vi "Read Core OOB TX.vi"(8 "error in (no error)":errorcluster, 11 "CIFCorePlugin in":refnum<class "CIFCorePlugin.lvclass">) -> (0 "error out":errorcluster, 3 "CIFCorePlugin out":refnum<class "CIFCorePlugin.lvclass">)   [LabVIEW 2021, in "CIFCorePlugin.lvclass"]
uses:
  CIFCorePlugin.lvclass
  CIFCorePlugin.lvclass/CIFCorePlugin.ctl
  Channels/CIFChannelMng/CIFChannelMng.lvclass/CIFChannelMng.ctl
  e064c0da-9abb-41e4-9ae5-21a8637ddf9c.vi
  Channels/CIFChannelMng/SubVIs/Read Channel List.vi
  Channels/CIFChannelMng/Core/Refresh Channel Data.vi/8bba354e-317d-4116-a685-ab5cd7060b87.vi
  <vilib>/CIF Foundation/CIF CIPC/SubVIs/Wait For N Elements Available.vi
  <vilib>/CIF Foundation/CIF CIPC/SubVIs/Check Error.vi
  <vilib>/CIF Foundation/CIF CIPC/SubVIs/Get dll Path.vi
  <vilib>/CIF Foundation/CIF CIPC/SubVIs/Get Element Read Position.vi
  <vilib>/CIF Foundation/CIF CIPC/SubVIs/Set Element Read Position.vi
  Utilities/Clocks/Update Clock.vi
  <vilib>/CIF Foundation/CIF CIPC/SubVIs/Get Element Info Variant.vi
  <vilib>/Utility/error.llb/Trim Whitespace.vi
  <vilib>/Utility/error.llb/Error Cluster From Error Code.vi
  CIFPluginManager/gRPC/CIF_Manager_Client_Wrapper/Internal/Update Clock.vi
  Channels/CIFChannelMng/CIFChannelMng.lvclass
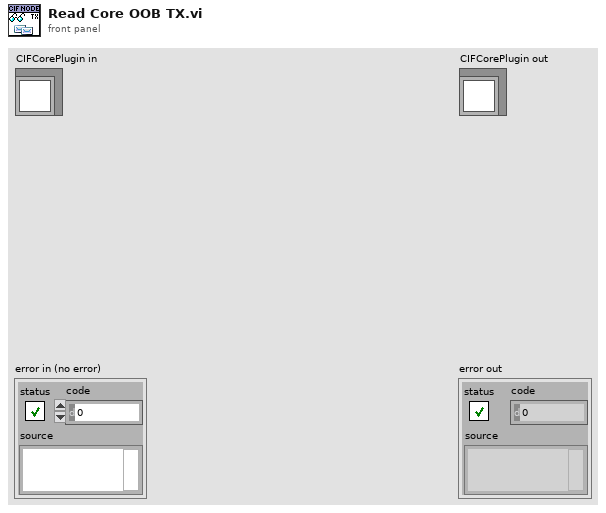
[diagram p1: front panel]
types:
  T1 = typedef "CIFCorePlugin.lvclass/Main to gRPC Data.ctl" = cluster{"Status":T2, "Plugin Overrides":T11, "External Time Source":T13}
  T2 = typedef "CIFCoreCommon.lvlib/Plugin Status.ctl" = cluster{"State":T3, "Timing Statistics (us)":T4, "FIFO Statistics (us)":T6, "error":T7, "Monitor Doubles":T8, "Monitor U64":T9, "Monitor I64":T10}
  T3 = typedef "CIFCoreCommon.lvlib/Plugin State.ctl" = enum32{"Null", "Creating", "Listening", "Running", "CleaningUp", "Destroying"}
  T4 = typedef "CIFCoreCommon.lvlib/Timing Statistics.ctl" = cluster{"Period":T5, "Wake Error":T5, "Execute":T5, "Housekeep":T5, "Idle":T5, "Cleanup":T5, "Custom 1 (custom units)":T5, "Custom 2 (custom units)":T5}
  T5 = typedef "CIFCoreCommon.lvlib/Timing Stats Base.ctl" = cluster{"Max":i64, "Avg":dbl, "Min":i64}
  T6 = typedef "CIFCoreCommon.lvlib/FIFO Statistics.ctl" = cluster{"From T0":T5, "From Previous Plugin":T5, "Output Error":T5}
  T7 = typedef "CIFCoreCommon.lvlib/Simple Error.ctl" = cluster{"status":bool, "code":i32}
  T8 = typedef "CIFCoreCommon.lvlib/Monitor Doubles.ctl" = cluster{"1":dbl, "2":dbl, "3":dbl, "4":dbl}
  T9 = typedef "CIFCoreCommon.lvlib/Monitor U64.ctl" = cluster{"1":u64, "2":u64, "3":u64, "4":u64}
  T10 = typedef "CIFCoreCommon.lvlib/Monitor I64.ctl" = cluster{"1":i64, "2":i64, "3":i64, "4":i64}
  T11 = typedef "CIFCoreCommon.lvlib/Plugin Overrides.ctl" = cluster{"Timing Overrides":T12}
  T12 = typedef "CIFCoreCommon.lvlib/Timing Overrides.ctl" = cluster{"Override Timing":bool, "Skip Sleep":bool, "Period (s)":dbl}
  T13 = typedef "CIFCoreCommon.lvlib/External Time Source.ctl" = cluster{"System Time":i64, "External Time":i64, "Counter":u64}
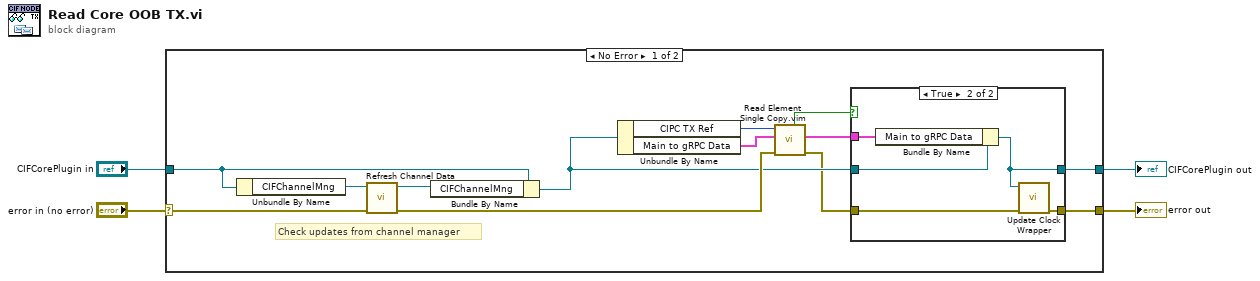
[diagram p0: block diagram]
diagram:
  n1 = case shown="No Error" "error in (no error)" {
    selector: "error in (no error)" -> [w14 w26]
    tunnel: [w5 w26] -> w3
    tunnel: [w17 w25] -> w1
    tunnel: "CIFCorePlugin in" -> [w11 w25]
    frame No Error {
      # "Check updates from channel manager"
      n2 = Unbundle By Name(w11) -> ("CIFChannelMng"=w15:refnum<class "CIFChannelMng.lvclass">)
      n3 = call "Refresh Channel Data.vi"("error in (no error)"=w14, "CIFChannelMng in"=w15) -> ("error out"=w13:errorcluster, "CIFChannelMng out"=w16:refnum<class "CIFChannelMng.lvclass">)  [unwired: 8 in]
      n4 = Bundle By Name(cluster=w11, "CIFChannelMng"=w16) -> (w12:refnum<class "CIFCorePlugin.lvclass">)
      n5 = Unbundle By Name(w12) -> ("CIPC TX Ref"=w10:u64, "Main to gRPC Data"=w9:T1)
      n6 = call "Read Element Single Copy.vim"("error in (no error)"=w13, "Data in"=w9, "CIPC Reference in"=w10) -> ("error out"=w6:errorcluster, "Data out"=w7:T1, "Success"=w8:bool)  [unwired: 4 in, 2 out]
      n7 = case shown="True" w8 {
        tunnel: [w19 w20] -> w17
        tunnel: w12 -> [w19 w24]
        tunnel: w7 -> [_ w23]
        tunnel: w6 -> [w18 w22]
        tunnel: [w18 w21] -> w5
        frame False {
        }
        frame True {
          n8 = Bundle By Name(cluster=w24, "Main to gRPC Data"=w23) -> (w20:refnum<class "CIFCorePlugin.lvclass">)
          n9 = call "Update Clock Wrapper.vi"("error in (no error)"=w22, "CIFCorePlugin in"=w20) -> ("error out"=w21:errorcluster)  [unwired: 9 in]
        }
      }
    }
    frame Error {
    }
  }
  "error out" <- w3
  "CIFCorePlugin out" <- w1
